vi "AKIP_write.vi"(8 "error in (no error)":errorcluster, 10 "write buffer":string, 11 "VISA Refnum in":refnum<visa-resource-name>="AKIP") -> (0 "error out":errorcluster, 3 "VISA Refnum out":refnum<visa-resource-name>)   [LabVIEW 2017]
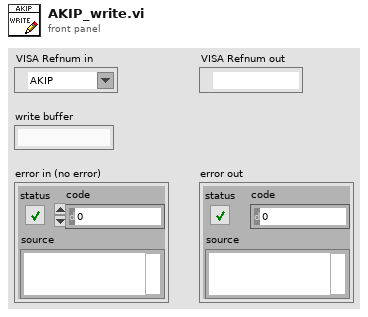
[diagram p1: front panel]
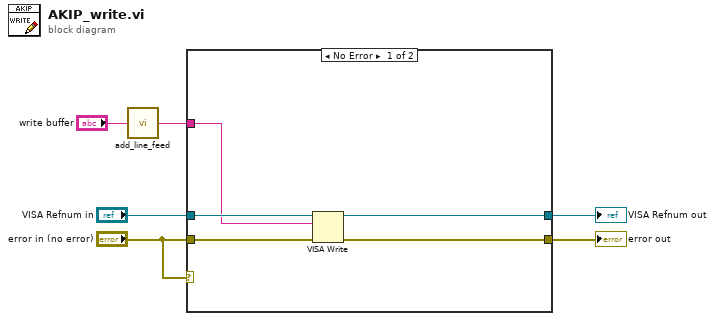
[diagram p0: block diagram]
diagram:
  n1 = call "add_line_feed.vi"("Input string"="write buffer") -> ("Output string"=w1:string)
  n2 = case shown="No Error" "error in (no error)" {
    tunnel: "error in (no error)" -> [w11 w12]
    tunnel: "VISA Refnum in" -> [w10 w13]
    tunnel: [w7 w12] -> w5
    tunnel: [w8 w13] -> w4
    tunnel: w1 -> [w9 _]
    frame No Error {
      n3 = VISA Write(VISA resource name=w10, write buffer=w9, error in (no error)=w11) -> (VISA resource name out=w8:refnum<visa-resource-name>, error out=w7:errorcluster)  [unwired: 1 out]
    }
    frame Error {
    }
  }
  "error out" <- w5
  "VISA Refnum out" <- w4
